vi "Dilate_Low_Auto.vi"(4 "Error IN Toolkit":i32, 5 "Error IN LabVIEW":errorcluster, 6 "Radio":i32) -> (18 "Error OUT Toolkit":i32, 19 "Error OUT LabVIEW":errorcluster)   [LabVIEW 2018]
doc: "\"Dilate\" is the opposite of \"Erode\". Here, a pixel element is '1' if at least one pixel of the image of those falling inside the kernel (radio) window is '1'. Therefore, Dilate increases the size of the foreground objects, that is, the white region. It receives the radio known as the kernel, which is the checking area.\n\nFor correct operation it should receive an error that comes from a VI of some processing algorithm or that contains a copy data of CPU-GPU."
uses:
  dll/LibreriaAutis_3.dll
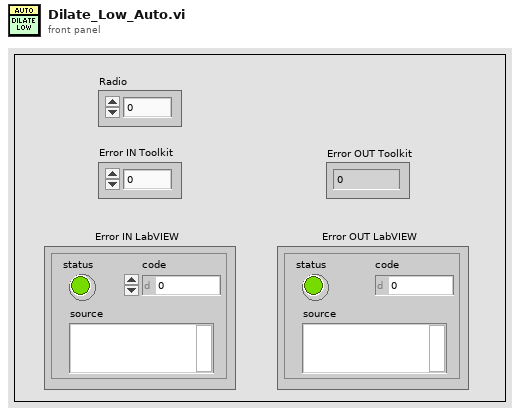
[diagram p1: front panel]
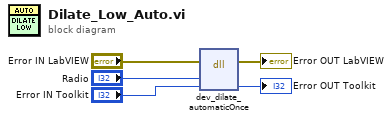
[diagram p0: block diagram]
diagram:
  n1 = dll-call lib="C:/Users/AUTIS/Desktop/LibreriaAUTIS/LabVIEW/dll/LibreriaAutis_3.dll" fn="dev_dilate_automaticOnce"(error in="Error IN LabVIEW", "radio"="Radio", "error"="Error IN Toolkit") -> (error out=→"Error OUT LabVIEW":errorcluster, "error"=→"Error OUT Toolkit":i32)  [unwired: 4 in, 1 out]
